vi "Parse Tx Generic Frame.vi"(8 "error in":errorcluster, 11 "node in":refnum<k20>) -> (0 "error out":errorcluster, 3 "Frame Generic":T1 {"Parameters"."Parameter"."encoding" items=["BNR", "BCD", "Discrete"]; "Frame header"."SequenceNumberOffset" items=["FDX_TX_FRAME_SEQ_OFFS_AUTO"=65535]; "Frame header"."SequenceNumberInit" items=["FDX_TX_FRAME_SEQ_INIT_AUTO"=65535, "FDX_TX_FRAME_SEQ_OFF"=65533]; "Frame header"."PhysErrorInjection" items=["FDX_TX_FRAME_ERR_OFF", "FDX_TX_FRAME_ERR_CRC", "FDX_TX_FRAME_ERR_ALI", "FDX_TX_FRAME_ERR_PRE", "FDX_TX_FRAME_ERR_PHY"]; "Frame header"."PayloadGenerationMode" items=["FDX_TX_FRAME_PGM_USER", "FDX_TX_FRAME_PGM_IP_PART", "FDX_TX_FRAME_PGM_IP_PART_TT", "FDX_TX_FRAME_PGM_IP_FULL", "FDX_TX_FRAME_PGM_IP_FULL_TT"]; "Frame header"."PayloadBufferMode" items=["FDX_TX_FRAME_PBM_STD", "FDX_TX_FRAME_PBM_MAC", "FDX_TX_FRAME_PBM_UDP", "FDX_TX_FRAME_PBM_FULL"]; "Frame header"."NetSelect" items=["FDX_TX_FRAME_DLY_A"=0, "FDX_TX_FRAME_DLY_B"=1, "FDX_TX_FRAME_BOTH "=3, "FDX_TX_FRAME_ONLY_A"=4, "FDX_TX_FRAME_ONLY_B "=5]; "Frame header"."FrameStartMode" items=["FDX_TX_FRAME_START_IFG", "FDX_TX_FRAME_START_PGWT", "FDX_TX_FRAME_START_TRG", "FDX_TX_FRAME_START_TRG_D"]})   [LabVIEW 2020, in "AIM ARINC 664 Import.lvlib"]
uses:
  AIM ARINC 664 Import.lvlib
  _typedefs/frame_tx_generic.ctl
  _typedefs/frame_tx_generic_seqNumberOffset.ctl
  _typedefs/frame_tx_generic_seqNumberInit.ctl
  _typedefs/frame_parameter_definition.ctl
  _typedefs/frame_parameter.ctl
  Shared/Encoding (Arinc664).ctl
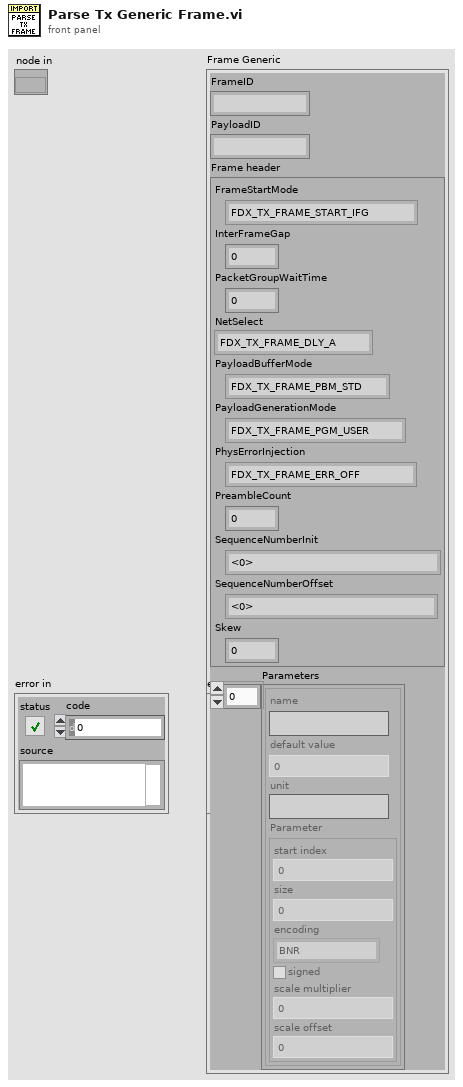
[diagram p1: front panel]
types:
  T1 = typedef "AIM ARINC 664 Import.lvlib/frame_tx_generic.ctl" = cluster{"FrameID":string, "PayloadID":string, "Frame header":cluster{"FrameStartMode":i32, "InterFrameGap":i32, "PacketGroupWaitTime":i32, "NetSelect":u32, "PayloadBufferMode":i32, "PayloadGenerationMode":i32, "PhysErrorInjection":i32, "PreambleCount":i32, "SequenceNumberInit":T2, "SequenceNumberOffset":T3, "Skew":i32}, "Parameters":T4[]}
  T2 = typedef "AIM ARINC 664 Import.lvlib/frame_tx_generic_seqNumberInit.ctl" = i32
  T3 = typedef "AIM ARINC 664 Import.lvlib/frame_tx_generic_seqNumberOffset.ctl" = i32
  T4 = typedef "AIM ARINC 664 Import.lvlib/frame_parameter.ctl" = cluster{"name":string, "default value":dbl, "unit":string, "Parameter":T5}
  T5 = typedef "AIM ARINC 664 Import.lvlib/frame_parameter_definition.ctl" = cluster{"start index":i32, "size":i32, "encoding":T6, "signed":bool, "scale multiplier":dbl, "scale offset":dbl}
  T6 = typedef "Encoding (Arinc664).ctl" = u16
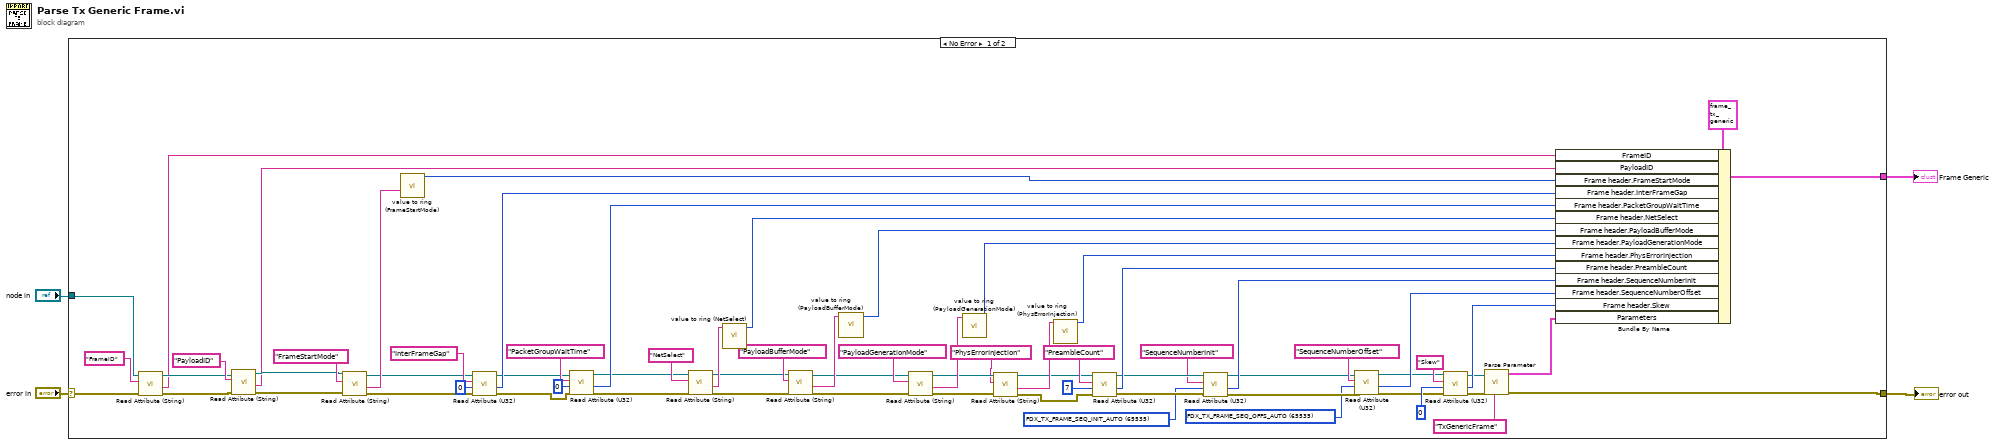
[diagram p0: block diagram]
diagram:
  n1 = case shown="No Error" "error in" {
    selector: "error in" -> [w14 w75]
    tunnel: "node in" -> [w11 _]
    tunnel: [w6 w75] -> w3
    tunnel: [w74 _] -> w1
    frame No Error {
      w19 = T3 65535 items=["FDX_TX_FRAME_SEQ_OFFS_AUTO"=65535] ("Frame header.SequenceNumberOffset")
      w23 = T2 65535 items=["FDX_TX_FRAME_SEQ_INIT_AUTO"=65535, "FDX_TX_FRAME_SEQ_OFF"=65533] ("Frame header.SequenceNumberInit")
      n2 = call "Read Attribute (String).vi"("error in"=w14, "Attribute Name"="FrameID" ("Tag Name"), "node in"=w11) -> ("error out"=w13:errorcluster, "value"=w10:string, "node out"=w12:refnum<k20>)  [unwired: 6 in]
      n3 = call "Read Attribute (String).vi"("error in"=w13, "Attribute Name"="PayloadID" ("Tag Name"), "node in"=w12) -> ("error out"=w65:errorcluster, "value"=w63:string, "node out"=w64:refnum<k20>)  [unwired: 6 in]
      n4 = call "Read Attribute (String).vi"("error in"=w65, "Attribute Name"="FrameStartMode" ("Name"), "node in"=w64) -> ("error out"=w73:errorcluster, "value"=w61:string, "node out"=w29:refnum<k20>)  [unwired: 6 in]
      n5 = call "value to ring (FrameStartMode).vi"("value"=w61) -> ("FrameStartMode"=w60:i32)  [unwired: 10 in]
      n6 = call "Read Attribute (U32).vi"("error in"=w73, "default"=u32 0, "Attribute Name"="InterFrameGap" ("Tag Name"), "node in"=w29) -> ("error out"=w56:errorcluster, "value"=w59:u32, "node out"=w28:refnum<k20>)  [unwired: 5 in]
      n7 = call "Read Attribute (U32).vi"("error in"=w56, "default"=u32 0, "Attribute Name"="PacketGroupWaitTime" ("Tag Name"), "node in"=w28) -> ("error out"=w52:errorcluster, "value"=w55:u32, "node out"=w53:refnum<k20>)  [unwired: 5 in]
      n8 = call "Read Attribute (String).vi"("error in"=w52, "Attribute Name"="NetSelect" ("Name"), "node in"=w53) -> ("error out"=w45:errorcluster, "value"=w51:string, "node out"=w46:refnum<k20>)  [unwired: 6 in]
      n9 = call "value to ring (NetSelect).vi"("value"=w51) -> ("NetSelect"=w50:u32)  [unwired: 10 in]
      n10 = call "Read Attribute (String).vi"("error in"=w45, "Attribute Name"="PayloadBufferMode" ("Name"), "node in"=w46) -> ("error out"=w42:errorcluster, "value"=w48:string, "node out"=w43:refnum<k20>)  [unwired: 6 in]
      n11 = call "value to ring (PayloadBufferMode).vi"("value"=w48) -> ("PayloadBufferMode"=w47:i32)  [unwired: 10 in]
      n12 = call "Read Attribute (String).vi"("error in"=w42, "Attribute Name"="PayloadGenerationMode" ("Name"), "node in"=w43) -> ("error out"=w37:errorcluster, "value"=w41:string, "node out"=w38:refnum<k20>)  [unwired: 6 in]
      n13 = call "value to ring (PayloadGenerationMode).vi"("value"=w41) -> ("PayloadGenerationMode"=w40:i32)  [unwired: 10 in]
      n14 = call "Read Attribute (String).vi"("error in"=w37, "Attribute Name"="PhysErrorInjection" ("Name"), "node in"=w38) -> ("error out"=w31:errorcluster, "value"=w35:string, "node out"=w32:refnum<k20>)  [unwired: 6 in]
      n15 = call "value to ring (PhysErrorInjection).vi"("value"=w35) -> ("PhysErrorInjection"=w39:i32)  [unwired: 10 in]
      n16 = call "Read Attribute (U32).vi"("error in"=w31, "default"=u32 7, "Attribute Name"="PreambleCount" ("Tag Name"), "node in"=w32) -> ("error out"=w25:errorcluster, "value"=w30:u32, "node out"=w27:refnum<k20>)  [unwired: 5 in]
      n17 = call "Read Attribute (U32).vi"("error in"=w25, "default"=w23, "Attribute Name"="SequenceNumberInit" ("Name"), "node in"=w27) -> ("error out"=w22:errorcluster, "value"=w24:u32, "node out"=w20:refnum<k20>)  [unwired: 5 in]
      n18 = call "Read Attribute (U32).vi"("error in"=w22, "default"=w19, "Attribute Name"="SequenceNumberOffset" ("Name"), "node in"=w20) -> ("error out"=w17:errorcluster, "value"=w18:u32, "node out"=w16:refnum<k20>)  [unwired: 5 in]
      n19 = call "Read Attribute (U32).vi"("error in"=w17, "default"=u32 0, "Attribute Name"="Skew" ("Tag Name"), "node in"=w16) -> ("error out"=w7:errorcluster, "value"=w62:u32, "node out"=w8:refnum<k20>)  [unwired: 5 in]
      n20 = call "Parse Parameter.vi"("error text in"="TxGenericFrame", "error in"=w7, "node in"=w8) -> ("error out"=w6:errorcluster, "parametesrs"=w5:T4[])  [unwired: 7 in]
      n21 = Bundle By Name(cluster=T1 {"FrameID"="", "PayloadID"="", "Frame header"={"FrameStartMode"=0, "InterFrameGap"=0, "PacketGroupWaitTime"=0, "NetSelect"=0, "PayloadBufferMode"=0, "PayloadGenerationMode"=0, "PhysErrorInjection"=0, "PreambleCount"=0, "SequenceNumberInit"=0, "SequenceNumberOffset"=0, "Skew"=0}, "Parameters"=[]} ("Frame Generic"), "FrameID"=w10, "PayloadID"=w63, "Frame header.FrameStartMode"=w60, "Frame header.InterFrameGap"=w59, "Frame header.PacketGroupWaitTime"=w55, "Frame header.NetSelect"=w50, "Frame header.PayloadBufferMode"=w47, "Frame header.PayloadGenerationMode"=w40, "Frame header.PhysErrorInjection"=w39, "Frame header.PreambleCount"=w30, "Frame header.SequenceNumberInit"=w24, "Frame header.SequenceNumberOffset"=w18, "Frame header.Skew"=w62, "Parameters"=w5) -> (w74:T1)
    }
    frame Error {
    }
  }
  "error out" <- w3
  "Frame Generic" <- w1
